vi "ST_parse_save_audit_response.vi"(6 "recordset_in":variant[][](array[variant]), 8 "error_in":errorcluster, 11 "command_nmb":u8) -> (0 "error_out":errorcluster, 3 "reference_data_to_PLC":u8[](array[numeric]))   [LabVIEW 2020]
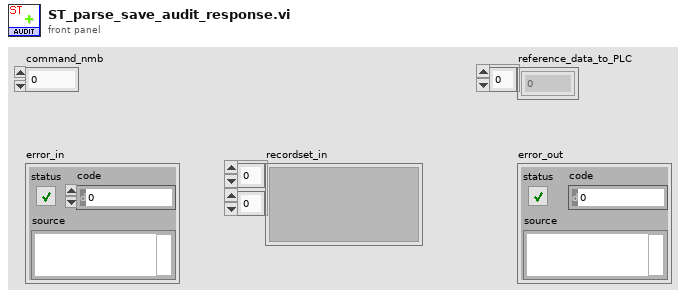
[diagram p1: front panel]
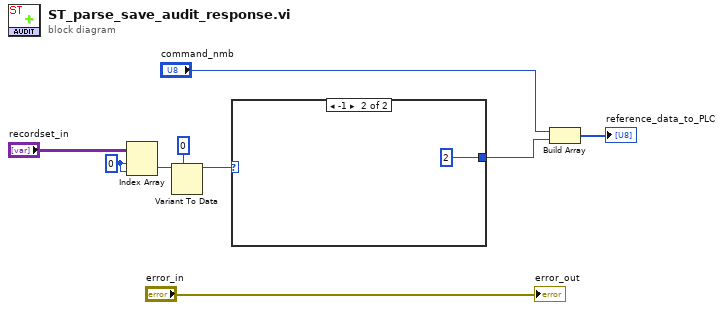
[diagram p0: block diagram]
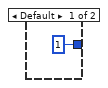
[diagram p2: hidden frame]
diagram:
  w4 = 0 ("index (row)")
  n1 = Index Array(array="recordset_in", index (row)=w4, index (col)=w4) -> (element=w3:variant)
  n2 = Variant To Data(type=0, Variant=w3) -> (data=w1:i32)  [unwired: 1 in, 1 out]
  n3 = case shown="-1" w1 {
    tunnel: [u8 1 u8 2] -> w7
    frame Default {
    }
    frame -1 {
    }
  }
  n4 = Build Array("command_nmb", w7) -> (→"reference_data_to_PLC":u8[])
  "error_out" <- "error_in"
